vi "Pump Data Mesuarement.vi"(8 "error in (no error)":errorcluster, 10 "Message Data":variant, 11 "Hardware Resources in":T1 {"Pump Info"."Direction" items=["CW", "CCW"]; "Pump Info"."Speed" format="%03.0f"}) -> (0 "error out":errorcluster, 1 "Contin":bool, 2 "Message Data Out":variant, 3 "Hardware Resources out":T1 {"Pump Info"."Direction" items=["CW", "CCW"]; "Pump Info"."Speed" format="%03.0f"})   [LabVIEW 2020, in "Pump.lvlib"]
doc: "Generates sample waveforms according to the signal type in the HW Config input."
uses:
  Pump.lvlib
  Pump Hardware Configuration.ctl
  support/Message Queue/Message Cluster.ctl
  support/HW Message Cluster.ctl
  support/Message Queue/Enqueue Message (Single).vi
  support/Message Queue/Message Queue.lvlib
  <instrlib>/WM Pump/WM Pump.lvlib
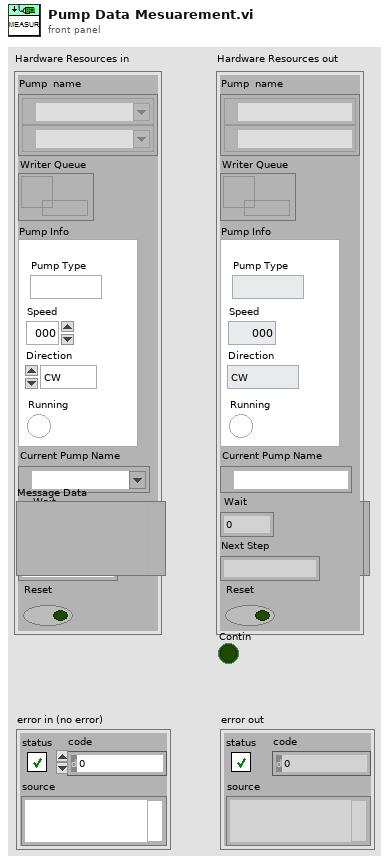
[diagram p1: front panel]
types:
  T1 = typedef "Pump.lvlib/Pump Hardware Configuration.ctl" = cluster{"Pump  name":refnum<visa-resource-name>[], "Writer Queue":refnum<queue>, "Pump Info":cluster{"Pump Type":string, "Speed":i32, "Direction":u16, "Running":bool}, "Current Pump Name":refnum<visa-resource-name>, "Wait":dbl, "Next Step":string, "Reset":bool}
  T2 = typedef "Message Queue.lvlib/HW Message Cluster.ctl" = cluster{"Writer Queue":refnum<queue>, "Writer Data":T3}
  T3 = typedef "Message Queue.lvlib/Message Cluster.ctl" = cluster{"Message":string, "Message Data":variant}
  T4 = cluster{"Pump Type":string, "Speed":i32, "Direction":u16, "Running":bool}
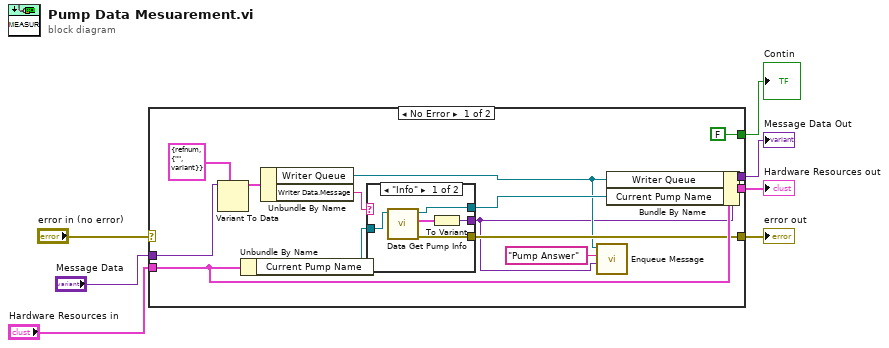
[diagram p0: block diagram]
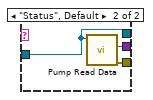
[diagram p2: hidden frame]
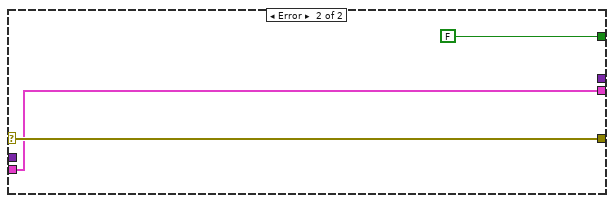
[diagram p3: hidden frame]
diagram:
  n1 = case shown="No Error" "error in (no error)" {
    selector: "error in (no error)" -> [_ w31]
    tunnel: [w13 w31] -> w6
    tunnel: [w8 _] -> w5
    tunnel: "Hardware Resources in" -> [w20 w30]
    tunnel: [w19 w30] -> w3
    tunnel: "Message Data" -> [w16 _]
    tunnel: [FALSE FALSE] -> w1
    frame No Error {
      n2 = Variant To Data(type=T2 {"Writer Queue"=refnum, "Writer Data"={"Message"="", "Message Data"=variant}}, Variant=w16) -> (data=w17:T2)  [unwired: 1 in, 1 out]
      n3 = Unbundle By Name(w20) -> ("Current Pump Name"=w14:refnum<visa-resource-name>)
      n4 = Unbundle By Name(w17) -> ("Writer Queue"=w10:refnum<queue>, "Writer Data.Message"=w12:string)
      n5 = case shown="\"Info\"" w12 {
        tunnel: [w23 w27] -> w15
        tunnel: w14 -> [w24 w27]
        tunnel: [w21 w26] -> w13
        tunnel: [w25 w28] -> w8
        frame "Info" {
          n6 = call <instrlib>:"Data Get Pump Info.vi"("VISA resource name"=w24) -> ("error out"=w21:errorcluster, "Pump Info"=w22:T4, "VISA resource name out"=w23:refnum<visa-resource-name>)  [unwired: 8 in]
          n7 = To Variant(anything=w22) -> (Variant=w25:variant)
        }
        frame "Status", Default {
          n8 = call "Pump Read Data.vi"("VISA Refnum in"=w27) -> ("error out"=w26:errorcluster, "Variant"=w28:variant)  [unwired: 9 in]
        }
      }
      n9 = call-poly "Enqueue Message.vi"("Message Data"=w8, "Message"="Pump Answer", "Message Queue"=w10) -> ()  [unwired: 7 in, 2 out]
      n10 = Bundle By Name(cluster=w20, "Writer Queue"=w10, "Current Pump Name"=w15) -> (w19:T1)
    }
    frame Error {
    }
  }
  "error out" <- w6
  "Message Data Out" <- w5
  "Hardware Resources out" <- w3
  "Contin" <- w1
